vi "GetAliasNames.vi"(0 "reference in":refnum<class "SwitchBase.lvclass">, 5 "error in (no error)":errorcluster) -> (14 "reference in":refnum<class "SwitchBase.lvclass">, 16 "Names":string[](array[string]), 19 "error out":errorcluster)   [LabVIEW 2017]
uses:
  SwitchBase.lvclass
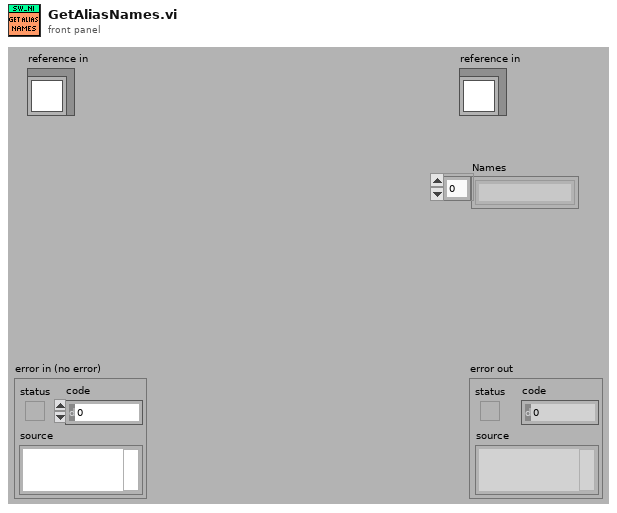
[diagram p1: front panel]
types:
  T1 = typedef "SwitchBase.lvlib/SwitchBase.lvclass/ObjectAttributes.ctl" = cluster{"Config":T2, "History":string[], "channel 1":string, "channel 2":string, "ActiveAlias":string, "AliasState":bool}
  T2 = typedef "SwitchBase.lvlib/SwitchBase.lvclass/Config.ctl" = cluster{"Resource":refnum<k15>, "topology name":T3, "Alias":cluster{"Name":string, "C1,C2":string[][]}[]}
  T3 = typedef "niSwitch Topologies.ctl" = string
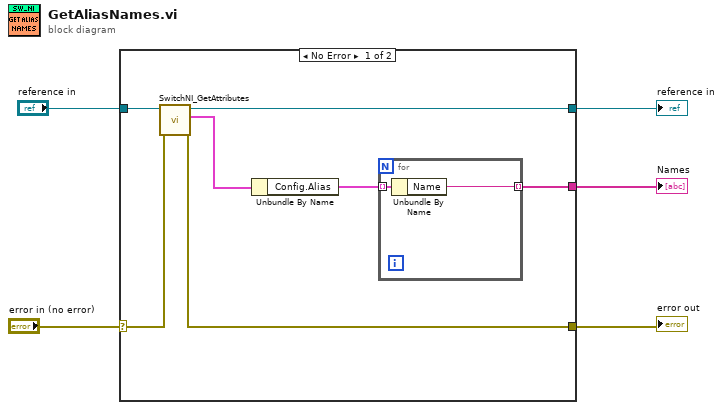
[diagram p0: block diagram]
diagram:
  n1 = case shown="No Error" "error in (no error)" {
    selector: "error in (no error)" -> [w12 w16]
    tunnel: [w10 w16] -> w4
    tunnel: [w8 w15] -> w2
    tunnel: "reference in" -> [w9 w15]
    tunnel: [w6 _] -> w1
    frame No Error {
      n2 = call "SwitchNI_GetAttributes.vi"("error in (no error)"=w12, "reference in"=w9) -> ("error out"=w10:errorcluster, "Data"=w11:T1, "reference out"=w8:refnum<class "SwitchBase.lvclass">)  [unwired: 6 in, 1 out]
      n3 = Unbundle By Name(w11) -> ("Config.Alias"=w7:cluster{"Name":string, "C1,C2":string[][]}[])
      n4 = for {
        tunnel: w7 -> [w14] mode=indexing
        tunnel: [w13] -> w6 mode=indexing
        n5 = Unbundle By Name(w14) -> ("Name"=w13:string)
      }
    }
    frame Error {
    }
  }
  "error out" <- w4
  "reference in" <- w2
  "Names" <- w1
